vi "subFindTargetsWithBuildSpec.vi"(8 "error in (no error)":errorcluster, 10 "Build Spec Name":string, 11 "Project":path) -> (0 "error out":errorcluster, 1 "Targets with spec name":string[](array[string]), 2 "dup Build Spec Name":string, 3 "dup Project":path)   [LabVIEW 2016, in "lvcommonbuild.lvlib"]
uses:
  lvcommonbuild.lvlib
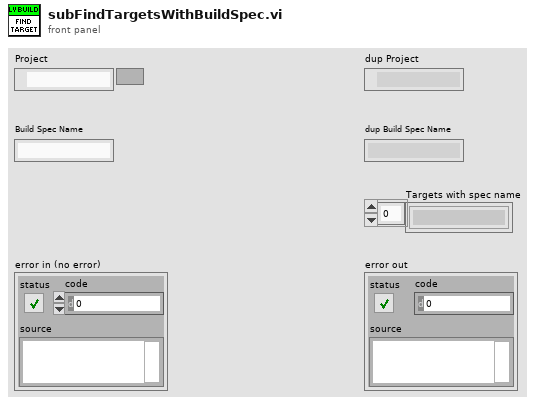
[diagram p1: front panel]
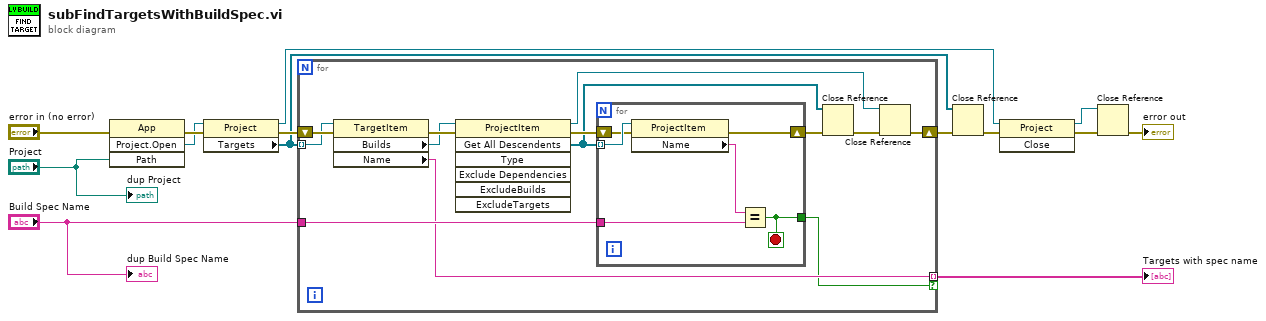
[diagram p0: block diagram]
diagram:
  n1 = invoke class="App" method="Project.Open"(error in="error in (no error)", "Path"="Project") -> (error out=w12:errorcluster, "Project:Open"=w11:refnum<vi>)  [unwired: 2 in, 2 out]
  n2 = property class="Project"(reference=w11, error in=w12) -> (reference out=w3:refnum<vi>, error out=w10:errorcluster, "Targets"=w5:refnum<vi>[])
  n3 = for {
    tunnel: w5 -> [w26] mode=indexing
    shift-right: [w16] -> w7
    shift-left: w10 -> [w27]
    tunnel: "Build Spec Name" -> [w22]
    tunnel: [w20] -> w8 mode=indexing if=w19
    n4 = property class="TargetItem"(reference=w26, error in=w27) -> (error out=w25:errorcluster, "Builds"=w24:refnum<vi>, "Name"=w20:string)  [unwired: 1 out]
    n5 = invoke class="ProjectItem" method="Get All Descendents"(reference=w24, error in=w25) -> (reference out=w15:refnum<vi>, error out=w23:errorcluster, "All Descendents"=w17:refnum<vi>[])  [unwired: 5 in, 4 out]
    n6 = for {
      tunnel: w17 -> [w33] mode=indexing
      shift-right: [w28] -> w21
      shift-left: w23 -> [w32]
      tunnel: w22 -> [w30]
      tunnel: [w29] -> w19
      stop <- w29 stop-if-true
      n7 = property class="ProjectItem"(reference=w33, error in=w32) -> (error out=w28:errorcluster, "Name"=w31:string)  [unwired: 1 out]
      n8 = Equal?(x=w31, y=w30) -> (x = y?=w29:bool)
    }
    n9 = Close Reference(reference=w17, error in (no error)=w21) -> (error out=w18:errorcluster)
    n10 = Close Reference(reference=w15, error in (no error)=w18) -> (error out=w16:errorcluster)
  }
  "Targets with spec name" <- w8
  n11 = Close Reference(reference=w5, error in (no error)=w7) -> (error out=w6:errorcluster)
  n12 = invoke class="Project" method="Close"(reference=w3, error in=w6) -> (reference out=w1:refnum<vi>, error out=w4:errorcluster)  [unwired: 1 in, 1 out]
  n13 = Close Reference(reference=w1, error in (no error)=w4) -> (error out=→"error out":errorcluster)
  "dup Build Spec Name" <- "Build Spec Name"
  "dup Project" <- "Project"
